vi "Change State.vi"(9 "Skip":i32, 10 "New State":T1, 11 "Constructor String Parser In":T2) -> (3 "Constructor String Parser":T2)   [LabVIEW 2020, in "Stream.lvlib" / "URLPattern.lvclass"]
uses:
  URLPattern.lvclass
  Constructor String Parser.ctl
  Token.ctl
  Token Type.ctl
  URL Pattern Init.ctl
  Parser State.ctl
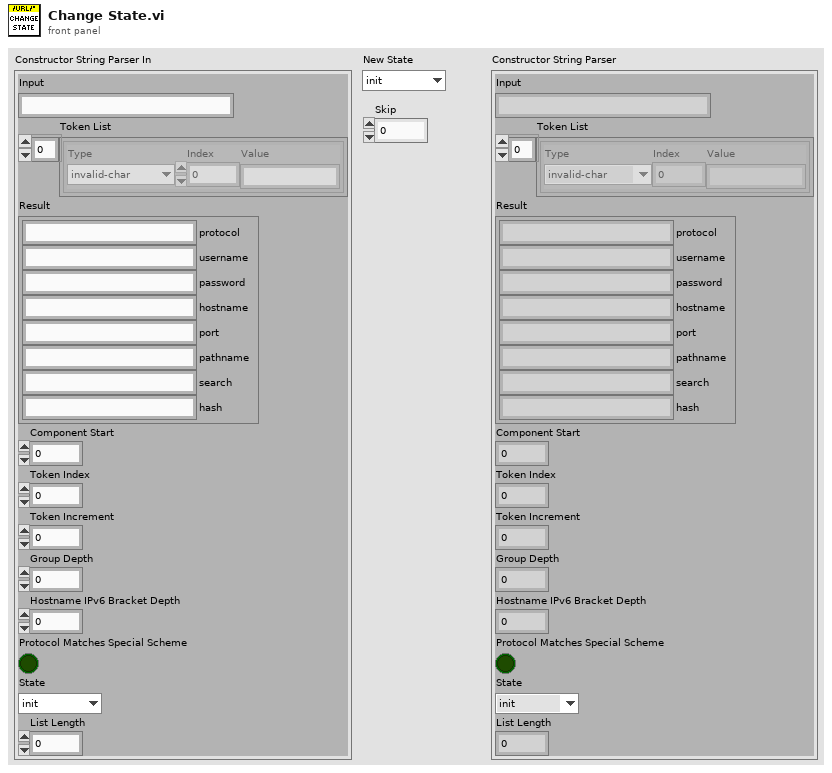
[diagram p1: front panel]
types:
  T1 = typedef "Stream.lvlib/URLPattern.lvclass/Parser State.ctl" = enum16{"init", "protocol", "authority", "username", "password", "hostname", "port", "pathname", "search", "hash", "done"}
  T2 = typedef "Stream.lvlib/URLPattern.lvclass/Constructor String Parser.ctl" = cluster{"Input":string, "Token List":T3[], "Result":T5, "Component Start":i32, "Token Index":i32, "Token Increment":i32, "Group Depth":i32, "Hostname IPv6 Bracket Depth":i32, "Protocol Matches Special Scheme":bool, "State":T1, "List Length":i32}
  T3 = typedef "Stream.lvlib/URLPattern.lvclass/Token.ctl" = cluster{"Type":T4, "Index":i32, "Value":string}
  T4 = typedef "Stream.lvlib/URLPattern.lvclass/Token Type.ctl" = enum16{"invalid-char", "open", "close", "regexp", "name", "char", "escaped-char", "other-modifier", "asterisk", "end"}
  T5 = typedef "Stream.lvlib/URLPattern.lvclass/URL Pattern Init.ctl" = cluster{"protocol":string, "username":string, "password":string, "hostname":string, "port":string, "pathname":string, "search":string, "hash":string}
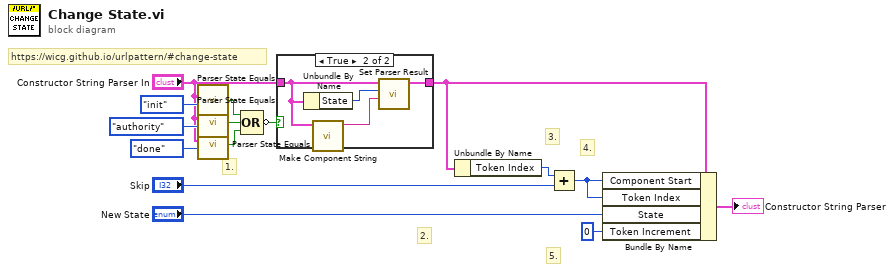
[diagram p0: block diagram]
diagram:
  # "https://wicg.github.io/urlpattern/#change-state"
  # "5."
  # "4."
  # "3."
  # "2."
  # "1."
  n1 = call "Parser State Equals.vi"("State"=Parser_State."init", "Constructor String Parser"="Constructor String Parser In") -> ("State Equals?"=w12:bool)  [unwired: 2 in]
  n2 = call "Parser State Equals.vi"("State"=Parser_State."authority", "Constructor String Parser"="Constructor String Parser In") -> ("State Equals?"=w11:bool)  [unwired: 2 in]
  n3 = call "Parser State Equals.vi"("State"=Parser_State."done", "Constructor String Parser"="Constructor String Parser In") -> ("State Equals?"=w10:bool)  [unwired: 2 in]
  n4 = Compound Arithmetic op=OR(w12, w11, w10) -> (invert w9:bool)
  n5 = case shown="True" w9 {
    tunnel: "Constructor String Parser In" -> [w16 w19]
    tunnel: [w16 w17] -> w6
    frame False {
    }
    frame True {
      n6 = Unbundle By Name(w19) -> ("State"=w18:T1)
      n7 = call "Make Component String.vi"("Constructor String Parser"=w19) -> ("Component String"=w20:string)  [unwired: 9 in, 1 out]
      n8 = call "Set Parser Result.vi"("Result"=w20, "State"=w18, "Constructor String Parser In"=w19) -> ("Constructor String Parser"=w17:T2)  [unwired: 8 in]
    }
  }
  n9 = Unbundle By Name(w6) -> ("Token Index"=w5:i32)
  n10 = Add(x=w5, y="Skip") -> (x+y=w3:i32)
  n11 = Bundle By Name(cluster=w6, "Component Start"=w3, "Token Index"=w3, "State"="New State", "Token Increment"=0) -> (→"Constructor String Parser":T2)
